vi "Save Signature Wizard Settings.vi"(0 "file path (use dialog)":path, 2 "Signature Analyzer Wizard Settings":T2={"Signature Description"="", "Start Connection"="", "Stop Connection"="", "Clock Connection"="", "Start POS"=FALSE, "Stop POS"=FALSE, "Clock POS"=FALSE, "NOP mode"=FALSE, "Enable Address Counter"=FALSE, "Force R/W to LOW (write)"=FALSE, "Connect SA START to A15"=FALSE, "Connect SA STOP to START"=FALSE, "Connect SA CLOCK to Phase2"=FALSE, "Notes"="", "Address Count Start"=0, "Address Count End"=65535, "Enable Data Counter"=FALSE, "Data Delay"=0, "Init Sequence"=[]} {"Init Sequence"."Data" format="%x"; "Init Sequence"."Address" format="%x"; "Address Count End" format="%04x"; "Address Count Start" format="%04x"}, 3 "Signature List":T1[](array[typedef]), 5 "error in":errorcluster) -> (19 "error out":errorcluster)   [LabVIEW 2018]
uses:
  Signature analyzer wizard settings.ctl
  Memory Read or Write Operation.ctl
  Init Operation.ctl
  Signature Definition.ctl
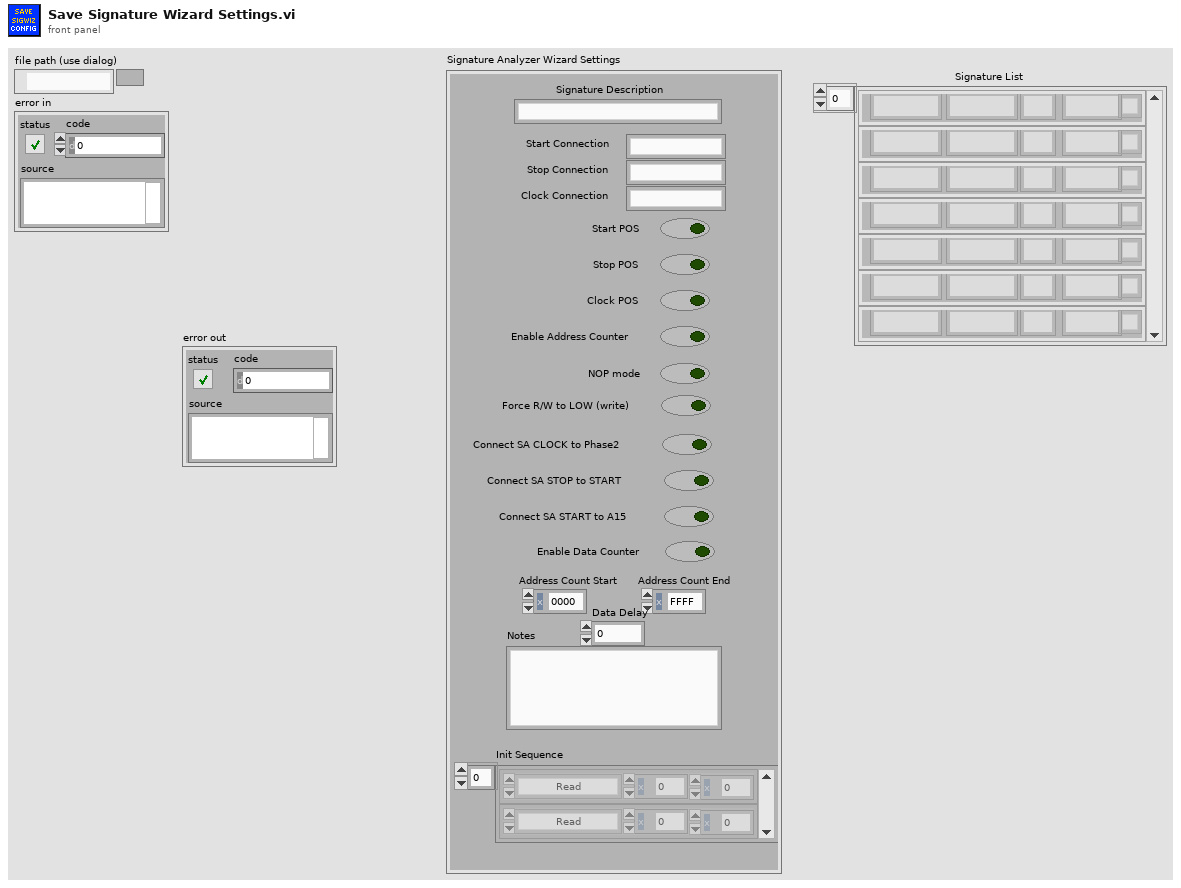
[diagram p1: front panel]
types:
  T1 = typedef "Signature Definition.ctl" = cluster{"Signal":string, "Location":string, "Pin":string, "Signature":string, " blank x or check":u16}
  T2 = typedef "Signature analyzer wizard settings.ctl" = cluster{"Signature Description":string, "Start Connection":string, "Stop Connection":string, "Clock Connection":string, "Start POS":bool, "Stop POS":bool, "Clock POS":bool, "NOP mode":bool, "Enable Address Counter":bool, "Force R/W to LOW (write)":bool, "Connect SA START to A15":bool, "Connect SA STOP to START":bool, "Connect SA CLOCK to Phase2":bool, "Notes":string, "Address Count Start":u16, "Address Count End":u16, "Enable Data Counter":bool, "Data Delay":u16, "Init Sequence":T3[]}
  T3 = typedef "Memory Read or Write Operation.ctl" = cluster{"Operation":T4, "Address":u16, "Data":u16}
  T4 = typedef "Init Operation.ctl" = enum16{"Read", "Write", "Compare", "IORead", "IOWrite", "IOCompare"}
  T5 = enum16{"open", "replace", "create", "open or create", "replace or create", "replace or create with confirmation"}
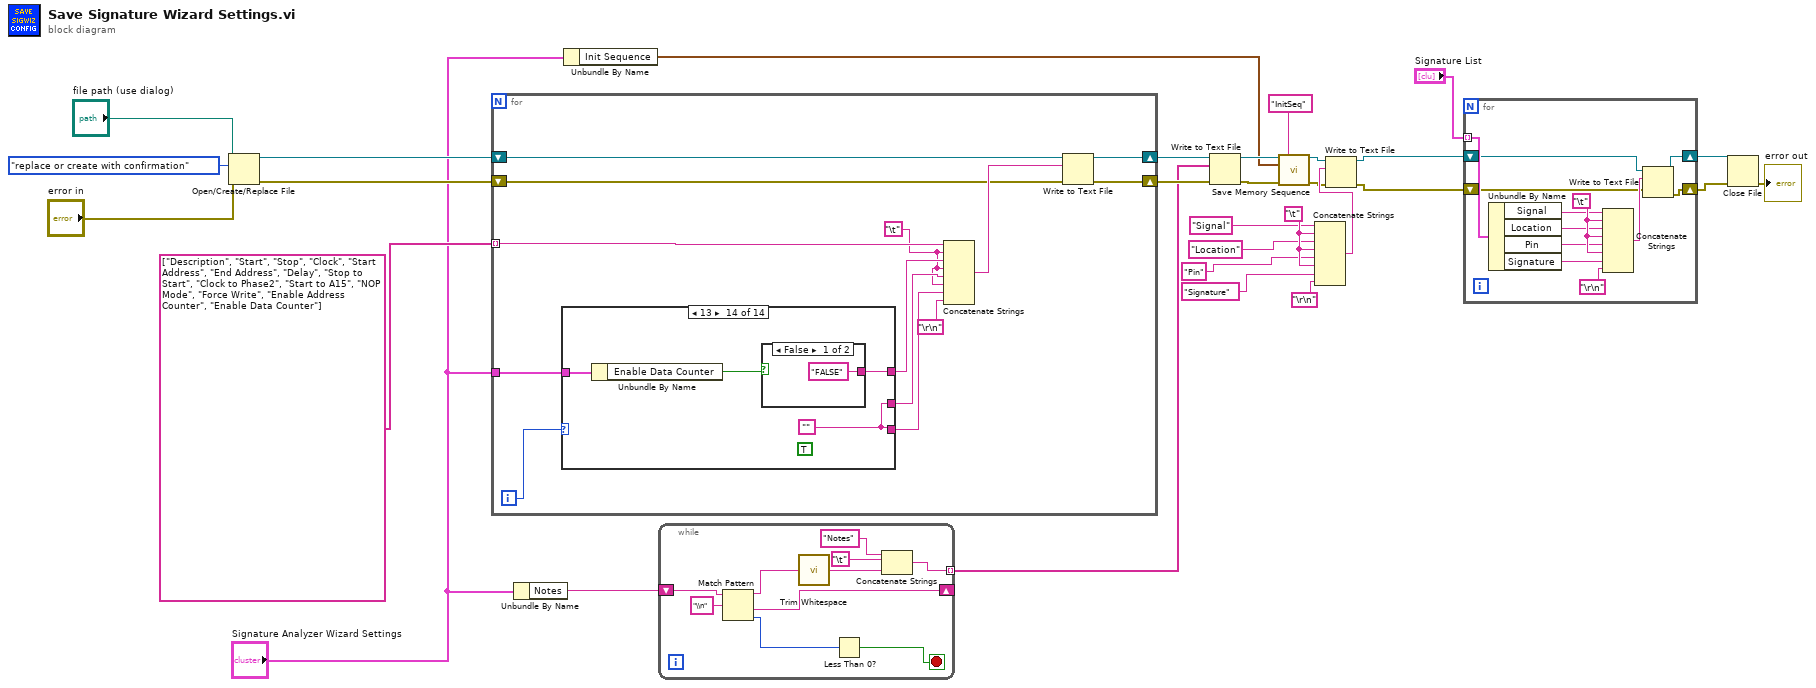
[diagram p0: block diagram]
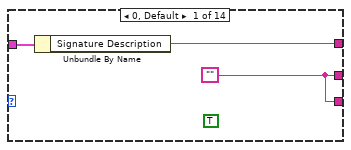
[diagram p2: hidden frame]
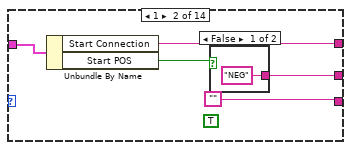
[diagram p3: hidden frame]
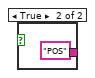
[diagram p4: hidden frame]
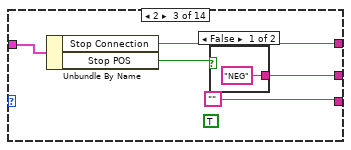
[diagram p5: hidden frame]
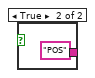
[diagram p6: hidden frame]
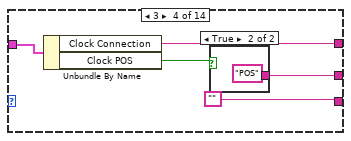
[diagram p7: hidden frame]
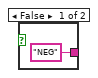
[diagram p8: hidden frame]
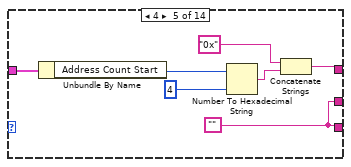
[diagram p9: hidden frame]
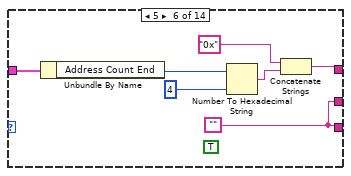
[diagram p10: hidden frame]
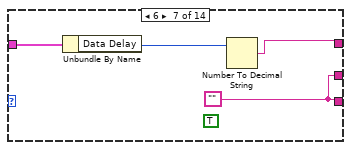
[diagram p11: hidden frame]
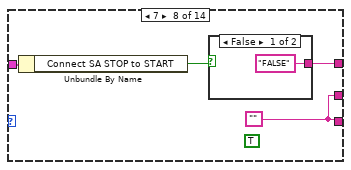
[diagram p12: hidden frame]
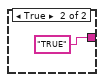
[diagram p13: hidden frame]
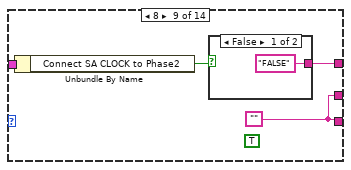
[diagram p14: hidden frame]
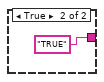
[diagram p15: hidden frame]
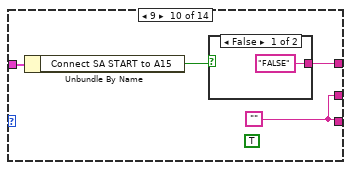
[diagram p16: hidden frame]
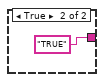
[diagram p17: hidden frame]
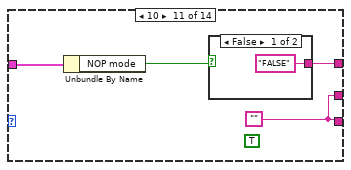
[diagram p18: hidden frame]
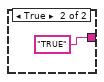
[diagram p19: hidden frame]
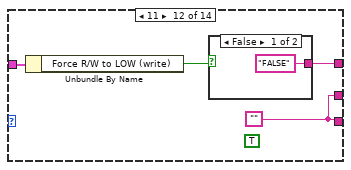
[diagram p20: hidden frame]
diagram:
  w13 = "\t"
  n1 = Open/Create/Replace File(file path (use dialog)="file path (use dialog)", error in="error in", operation (0:open)=T5."replace or create with confirmation") -> (refnum out=w26:refnum<file>, error out=w25:errorcluster)  [unwired: 3 in, 1 out]
  n2 = for {
    tunnel: string[] ["Description", "Start", "Stop", "Clock", "Start Address", "End Address", "Delay", "Stop to Start", "Clock to Phase2", "Start to A15", "NOP Mode", "Force Write", "Enable Address Counter", "Enable Data Counter"] -> [w42] mode=indexing
    shift-right: [w32] -> w23
    shift-left: w26 -> [w34]
    shift-right: [w31] -> w22
    shift-left: w25 -> [w33]
    tunnel: "Signature Analyzer Wizard Settings" -> [w41]
    i -> [w43]
    w38 = "\t"
    n3 = case shown="13" w43 {
      tunnel: w41 -> [w46 w51 w58 w65 w74 w81 w85 w89 w95 w101 w107 w113 w119 w125]
      tunnel: [w45 w50 w57 w64 w71 w78 w82 w87 w93 w99 w105 w111 w117 w123] -> w40
      tunnel: [w44 w47 w54 w61 w68 w75 w83 w88 w94 w100 w106 w112 w118 w124] -> w39
      tunnel: [w44 "" "" "" w68 w75 w83 w88 w94 w100 w106 w112 w118 w124] -> w37
      frame 0, Default {
        (unwired) TRUE
        w44 = ""
        n4 = Unbundle By Name(w46) -> ("Signature Description"=w45:string)
      }
      frame 1 {
        (unwired) TRUE
        n5 = Unbundle By Name(w51) -> ("Start Connection"=w50:string, "Start POS"=w48:bool)
        n6 = case shown="False" w48 {
          tunnel: ["NEG" "POS"] -> w47
          frame False {
          }
          frame True {
          }
        }
      }
      frame 2 {
        (unwired) TRUE
        n7 = Unbundle By Name(w58) -> ("Stop Connection"=w57:string, "Stop POS"=w55:bool)
        n8 = case shown="False" w55 {
          tunnel: ["NEG" "POS"] -> w54
          frame False {
          }
          frame True {
          }
        }
      }
      frame 3 {
        n9 = Unbundle By Name(w65) -> ("Clock Connection"=w64:string, "Clock POS"=w62:bool)
        n10 = case shown="True" w62 {
          tunnel: ["NEG" "POS"] -> w61
          frame False {
          }
          frame True {
          }
        }
      }
      frame 4 {
        w68 = ""
        n11 = Unbundle By Name(w74) -> ("Address Count Start"=w72:u16)
        n12 = Number To Hexadecimal String(1:i16 4 ("width (-)"), 2:w72) -> (0:w70:string)
        n13 = Concatenate Strings("0x" ("string"), w70) -> (w71:string)
      }
      frame 5 {
        (unwired) TRUE
        w75 = ""
        n14 = Unbundle By Name(w81) -> ("Address Count End"=w79:u16)
        n15 = Number To Hexadecimal String(1:i16 4 ("width (-)"), 2:w79) -> (0:w77:string)
        n16 = Concatenate Strings("0x" ("string"), w77) -> (w78:string)
      }
      frame 6 {
        (unwired) TRUE
        w83 = ""
        n17 = Unbundle By Name(w85) -> ("Data Delay"=w84:u16)
        n18 = Number To Decimal String(number=w84) -> (decimal integer string=w82:string)  [unwired: 1 in]
      }
      frame 7 {
        (unwired) TRUE
        w88 = ""
        n19 = Unbundle By Name(w89) -> ("Connect SA STOP to START"=w86:bool)
        n20 = case shown="False" w86 {
          tunnel: ["FALSE" "TRUE"] -> w87
          frame False {
          }
          frame True {
          }
        }
      }
      frame 8 {
        (unwired) TRUE
        w94 = ""
        n21 = Unbundle By Name(w95) -> ("Connect SA CLOCK to Phase2"=w92:bool)
        n22 = case shown="False" w92 {
          tunnel: ["FALSE" "TRUE"] -> w93
          frame False {
          }
          frame True {
          }
        }
      }
      frame 9 {
        (unwired) TRUE
        w100 = ""
        n23 = Unbundle By Name(w101) -> ("Connect SA START to A15"=w98:bool)
        n24 = case shown="False" w98 {
          tunnel: ["FALSE" "TRUE"] -> w99
          frame False {
          }
          frame True {
          }
        }
      }
      frame 10 {
        (unwired) TRUE
        w106 = ""
        n25 = Unbundle By Name(w107) -> ("NOP mode"=w104:bool)
        n26 = case shown="False" w104 {
          tunnel: ["FALSE" "TRUE"] -> w105
          frame False {
          }
          frame True {
          }
        }
      }
      frame 11 {
        (unwired) TRUE
        w112 = ""
        n27 = Unbundle By Name(w113) -> ("Force R/W to LOW (write)"=w110:bool)
        n28 = case shown="False" w110 {
          tunnel: ["FALSE" "TRUE"] -> w111
          frame False {
          }
          frame True {
          }
        }
      }
      frame 12 {
        (unwired) TRUE
        w118 = ""
        n29 = Unbundle By Name(w119) -> ("Enable Address Counter"=w116:bool)
        n30 = case shown="False" w116 {
          tunnel: ["FALSE" "TRUE"] -> w117
          frame False {
          }
          frame True {
          }
        }
      }
      frame 13 {
        (unwired) TRUE
        w124 = ""
        n31 = Unbundle By Name(w125) -> ("Enable Data Counter"=w122:bool)
        n32 = case shown="False" w122 {
          tunnel: ["FALSE" "TRUE"] -> w123
          frame False {
          }
          frame True {
          }
        }
      }
    }
    n33 = Concatenate Strings(w42, w38, w40, w38, w39, w38, w37, "\r\n") -> (w35:string)
    n34 = Write to Text File(file (use dialog)=w34, text=w35, error in=w33) -> (refnum out=w32:refnum<file>, error out=w31:errorcluster)  [unwired: 1 in, 1 out]
  }
  n35 = Unbundle By Name("Signature Analyzer Wizard Settings") -> ("Notes"=w24:string)
  n36 = Unbundle By Name("Signature Analyzer Wizard Settings") -> ("Init Sequence"=w1:T3[])
  n37 = while {
    shift-right: [w135] -> _
    shift-left: w24 -> [w136]
    tunnel: [w132] -> w21 mode=indexing
    stop <- w128 stop-if-true
    n38 = Match Pattern(string=w136, regular expression="\\n") -> (before substring=w134:string, after substring=w135:string, offset past match=w129:i32)  [unwired: 1 in, 1 out]
    n39 = call <vilib>:"Trim Whitespace.vi"("string"=w134) -> ("trimmed string"=w133:string)  [unwired: 1 in]
    n40 = Less Than 0?(x=w129) -> (x < 0?=w128:bool)
    n41 = Concatenate Strings("Notes" ("string"), "\t", w133) -> (w132:string)
  }
  n42 = Write to Text File(file (use dialog)=w23, text=w21, error in=w22) -> (refnum out=w4:refnum<file>, error out=w7:errorcluster)  [unwired: 1 in, 1 out]
  n43 = call "Save Memory Sequence.vi"("refnum in"=w4, "Token"="InitSeq", "Mem Sequence"=w1, "error in"=w7) -> ("refnum out"=w5:refnum<file>, "error out"=w6:errorcluster)  [unwired: 10 in]
  n44 = Concatenate Strings("Signal", w13, "Location", w13, "Pin", w13, "Signature", "\r\n") -> (w12:string)
  n45 = Write to Text File(file (use dialog)=w5, text=w12, error in=w6) -> (refnum out=w16:refnum<file>, error out=w15:errorcluster)  [unwired: 1 in, 1 out]
  n46 = for {
    tunnel: "Signature List" -> [w146] mode=indexing
    shift-right: [w139] -> w18
    shift-left: w15 -> [w140]
    shift-right: [w138] -> w19
    shift-left: w16 -> [w141]
    w148 = "\t"
    n47 = Unbundle By Name(w146) -> ("Signal"=w145:string, "Location"=w144:string, "Pin"=w143:string, "Signature"=w142:string)
    n48 = Concatenate Strings(w145, w148, w144, w148, w143, w148, w142, "\r\n") -> (w149:string)
    n49 = Write to Text File(file (use dialog)=w141, text=w149, error in=w140) -> (refnum out=w138:refnum<file>, error out=w139:errorcluster)  [unwired: 1 in, 1 out]
  }
  n50 = Close File(refnum=w19, error in=w18) -> (error out=→"error out":errorcluster)  [unwired: 1 out]
